vi "main.vi"() -> ()   [LabVIEW 2017]
uses:
  <vilib>/DAQmx/read.llb/DAQmx Read (Counter U32 1Chan 1Samp).vi
  <vilib>/DAQmx/write.llb/DAQmx Write (Digital 1D Bool 1Chan 1Samp).vi
  <vilib>/DAQmx/miscellaneous.llb/DAQmx Fill In Error Info.vi
panel:
  in  "Digital real/sham stim channels":tag="pciDAQ/port0/line1:2"
  in  "Analog pulse channel":tag="pciDAQ/ao0"
  in  "OEP sample clock in":tag="/pciDAQ/PFI0"
  in  "Onboard counter":tag="pciDAQ/ctr0"
  out "Learning rate (for adaptive threshold)":dbl(graph)
  out "Phase threshold":sgl(graph)
  in  "Stim even when\ntarget exceeded":bool=TRUE
  in  "Sham stimulations:":i32=1 min=0
  in  "Real stimulations:":i32=1 min=1
  out "Stim time":i64
  out "Crossing time":i64
  out "Crossing level":sgl
  out "Time on (samp.)":i64
  out "Clock offset":i64
  in  "OEP stim TTL chan":u16=4 caption="probe channel" min=1 max=8
  in  "event channel":u16=1 min=1 max=8
  in  "event port":u16=5557
  out "New event":bool
  in  "Max target":i64 min=0
  in  "Limit target":bool
  in  "Target delay":i64
  in  "Adapt target":bool
  out "Phase offset (deg.)":dbl
  in  "Avg signal freq (Hz)":dbl=6.0
  in  "Sample rate":dbl=30000.0
  in  "Stim enabled":bool
  out "OEP to LV delay":i64(graph)=402
  in  "Stop":bool
  # "*** Start OpenEphys acquisition before the VI. ***"
  # "*** In the audio settings in the OpenEphys GUI, reduce the buffer size to get a 10 ms buffer period.  If ASIO is installed and enabled in\nthe Open Ephys build, use ASIO with sample rate (in audio settings) = 192,000 Hz and buffer size = 192 (1 ms buffer period). ***"
  # "Inputs"
  # "Delay control"
  # "Stim pattern if enabled"
  # "Event info"
  # "Threshold estimation"
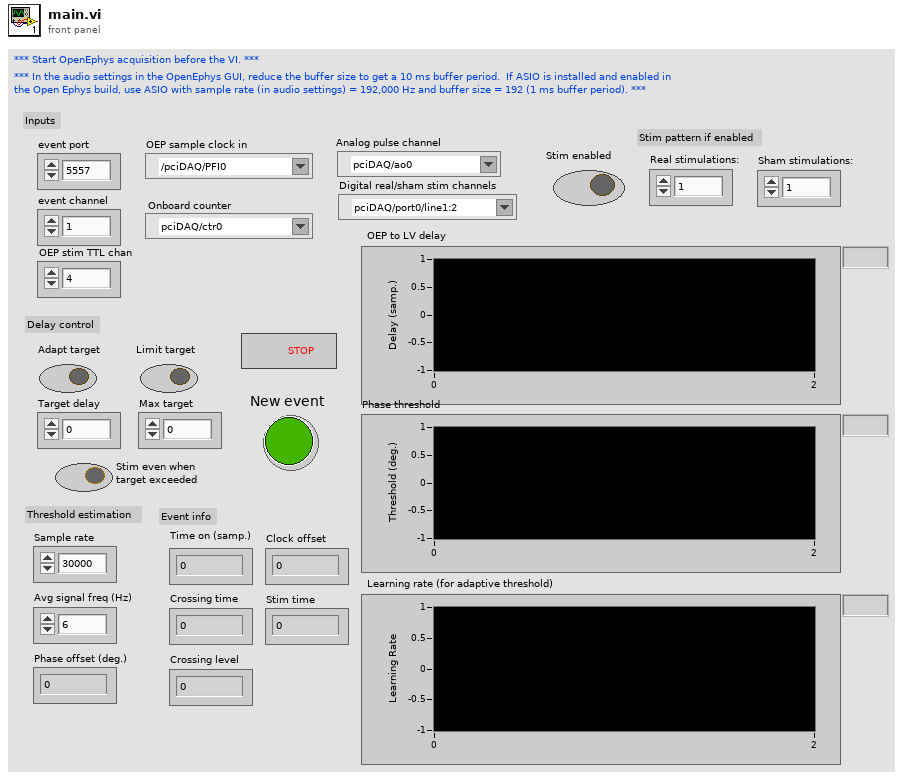
[diagram p1: front panel]
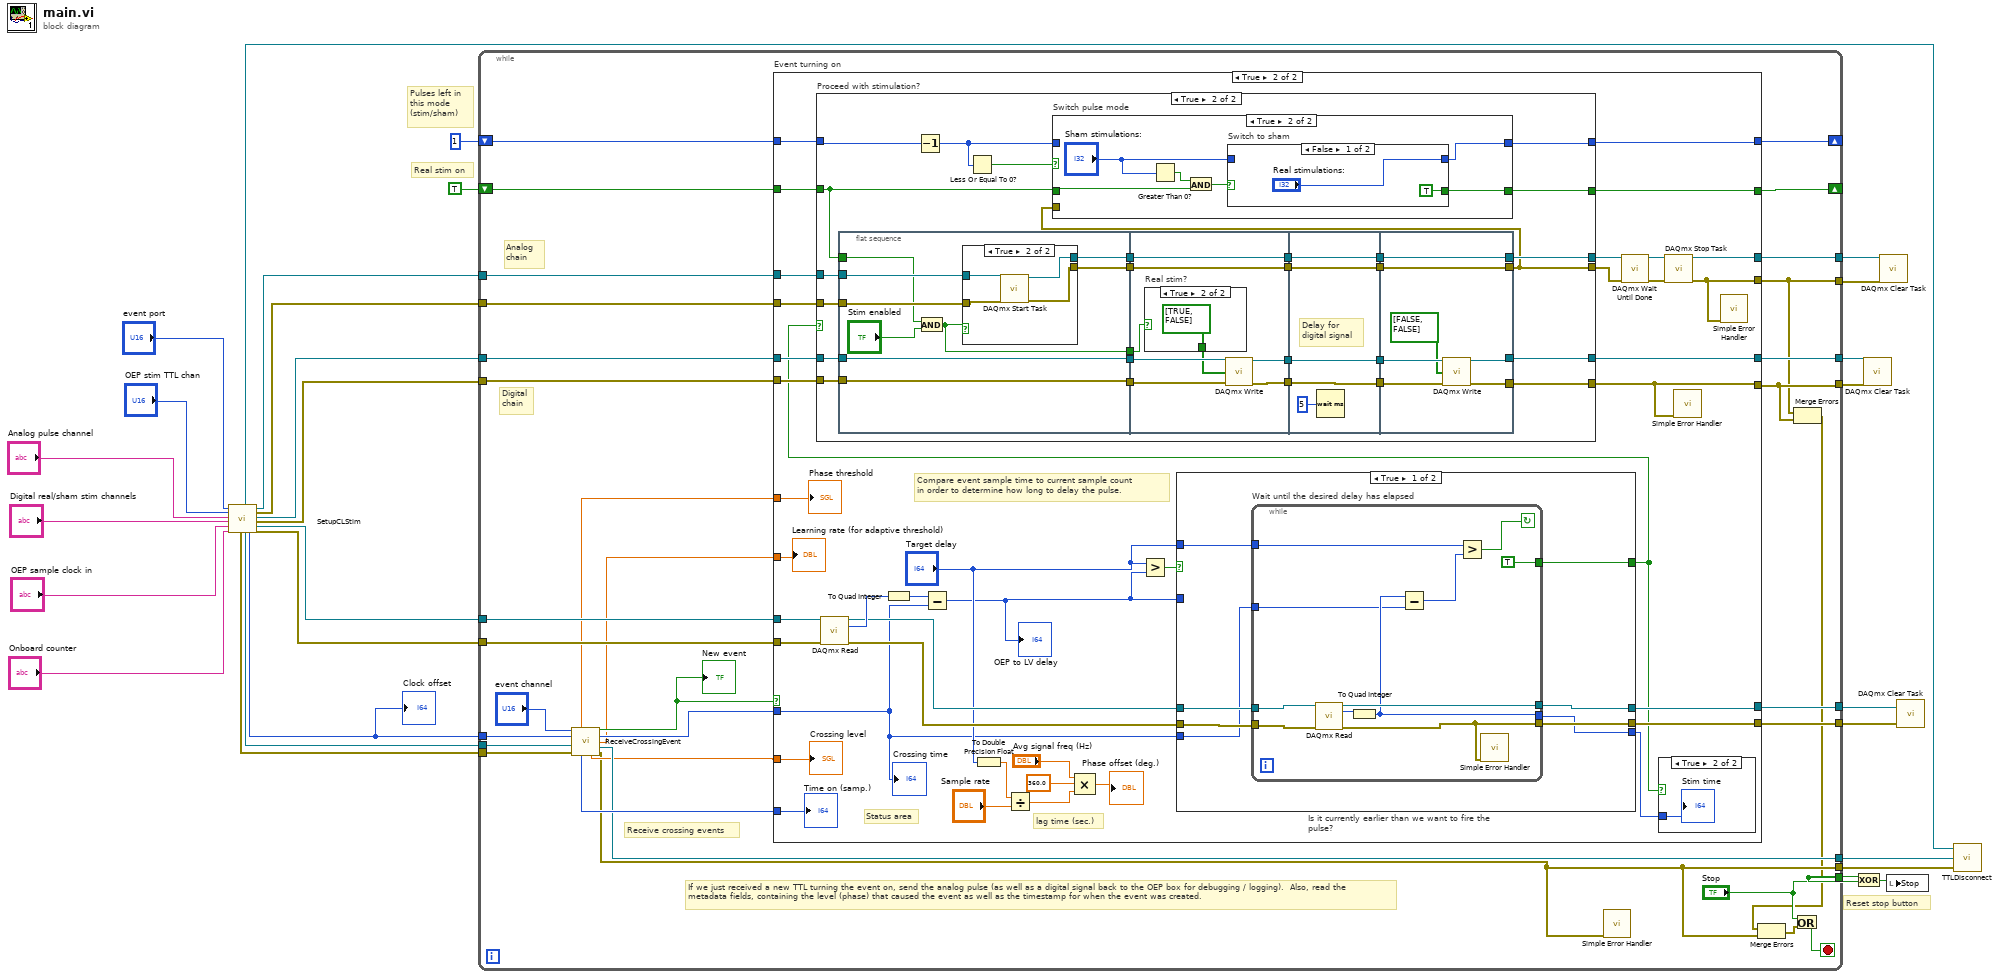
[diagram p0: block diagram]
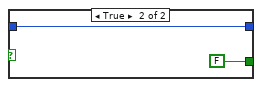
[diagram p6: hidden frame]
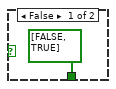
[diagram p8: hidden frame]
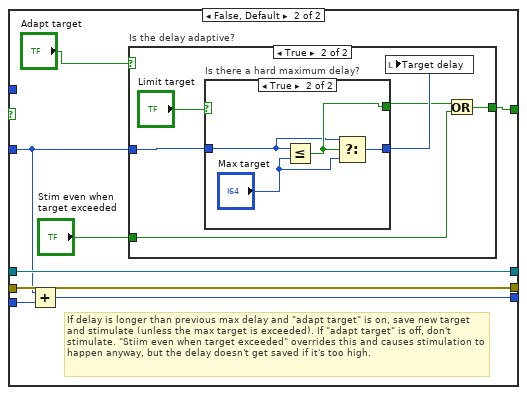
[diagram p9: hidden frame]
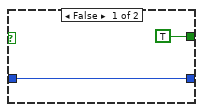
[diagram p11: hidden frame]
diagram:
  # "Pulses left in \nthis mode\n(stim/sham)"
  # "Real stim on"
  # "Reset stop button"
  n1 = call "SetupCLStim.vi"("event port"="event port", "OEP pulse channel"="OEP stim TTL chan", "Analog pulse channel"="Analog pulse channel", "Digital real/sham stim channels"="Digital real/sham stim channels", "OEP sample clock in"="OEP sample clock in", "Onboard counter"="Onboard counter") -> ("zmq error out"=w7:errorcluster, "context out"=w16:refnum<class "zmq_context.lvclass">, "socket out"=w8:refnum<class "zmq_socket.lvclass">, "clock offset"=w9:i64, "AO task out"=w15:refnum<k21>, "AO error out"=w14:errorcluster, "DO task out"=w13:refnum<k21>, "DO error out"=w12:errorcluster, "ctr task out"=w11:refnum<k21>, "ctr error out"=w10:errorcluster)  [unwired: 4 in]
  "Clock offset" <- w9
  n2 = while {
    tunnel: w7 -> [w49]
    tunnel: [w32] -> w24
    tunnel: w8 -> [w50]
    tunnel: w15 -> [w60]
    tunnel: w13 -> [w59]
    tunnel: w12 -> [w58]
    tunnel: w14 -> [w53]
    tunnel: [w51] -> w18
    tunnel: [w31] -> w17
    tunnel: [w57] -> w28
    tunnel: [w33] -> w27
    tunnel: ["Stop"] -> w26
    tunnel: w11 -> [w56]
    tunnel: [w55] -> w23
    tunnel: [w54] -> w22
    tunnel: w10 -> [w52]
    tunnel: [w45] -> w21
    shift-right: [w39] -> _
    shift-left: TRUE -> [w41]
    shift-right: [w40] -> _
    shift-left: 1 -> [w42]
    tunnel: w9 -> [w29]
    stop <- w36 stop-if-true
    # "Analog \nchain"
    # "Digital\nchain"
    # "If we just received a new TTL turning the event on, send the analog pulse (as well as a digital signal back to the OEP box for debugging / logging).  Also, read the metadata fields, containing the level (phase) that caused the event as well as the timestamp for when the event was created."
    # "Receive crossing events"
    n3 = call "ReceiveCrossingEvent.vi"("channel"="event channel", "clock offset"=w29, "socket in"=w50, "error in"=w49) -> ("threshold"=w38:sgl, "new crossing"=w48:bool, "crossing time"=w47:i64, "learning rate"=w37:dbl, "socket out"=w45:refnum<class "zmq_socket.lvclass">, "event time"=w46:i64, "crossing level"=w44:sgl, "error out"=w32:errorcluster)  [unwired: 3 in, 1 out]
    "New event" <- w48
    n4 = case "Event turning on" shown="True" w48 {
      tunnel: w60 -> [w68 w104]
      tunnel: w53 -> [w67 w103]
      tunnel: [w68 w95] -> w51
      tunnel: [w67 w72] -> w31
      tunnel: w59 -> [w66 w107]
      tunnel: w58 -> [w65 w105]
      tunnel: [w66 w108] -> w57
      tunnel: [w65 w71] -> w33
      tunnel: w47 -> [_ w90]
      tunnel: w56 -> [w64 w102]
      tunnel: w52 -> [w63 w99]
      tunnel: [w64 w97] -> w55
      tunnel: [w63 w96] -> w54
      tunnel: w46 -> [_ w91]
      tunnel: w44 -> [_ w85]
      tunnel: w42 -> [w62 w78]
      tunnel: w41 -> [w61 w77]
      tunnel: [w62 w76] -> w40
      tunnel: [w61 w75] -> w39
      tunnel: w38 -> [_ w74]
      tunnel: w37 -> [_ w73]
      frame False {
      }
      frame True {
        # "Status area"
        # "lag time (sec.)"
        # "Compare event sample time to current sample count\nin order to determine how long to delay the pulse."
        n5 = call-poly <vilib>:"DAQmx Read.vi"("task/channels in"=w102, "error in"=w99) -> ("task out"=w98:refnum<k21>, "data"=w101:u32, "error out"=w100:errorcluster)  [unwired: 11 in]
        n6 = To Quad Integer(1:w101) -> (0:w81:i64)
        n7 = Subtract(x=w81, y=w90) -> (x-y=w92:i64)
        "OEP to LV delay" <- w92
        n8 = To Double Precision Float(number="Target delay") -> (double precision float=w89:dbl)
        n9 = Divide(x=w89, y="Sample rate") -> (x/y=w88:dbl)
        n10 = Compound Arithmetic op=MULTIPLY("Avg signal freq (Hz)", 360.0 ("y"), w88) -> (→"Phase offset (deg.)":dbl)
        n11 = Greater?(x="Target delay", y=w92) -> (0:w106:bool)
        n12 = case "Is it currently earlier than we want to fire the pulse?" shown="True" w106 {
          tunnel: w92 -> [_ w213]
          tunnel: "Target delay" -> [w193 _]
          tunnel: w100 -> [w198 w218]
          tunnel: [w197 w218] -> w96
          tunnel: w90 -> [w192 w216]
          tunnel: w98 -> [w199 w217]
          tunnel: [w196 w217] -> w97
          tunnel: [w195 w212] -> w80
          tunnel: [w194 w215] -> w79
          frame True {
            n13 = while "Wait until the desired delay has elapsed" {
              tunnel: w199 -> [w209]
              tunnel: w198 -> [w210]
              tunnel: [w200] -> w197
              tunnel: [w208] -> w196
              tunnel: [TRUE] -> w195
              tunnel: [w203] -> w194
              tunnel: w193 -> [w204]
              tunnel: w192 -> [w202]
              stop <- w206 continue-if-true
              n14 = call-poly <vilib>:"DAQmx Read.vi"("task/channels in"=w209, "error in"=w210) -> ("task out"=w208:refnum<k21>, "data"=w205:u32, "error out"=w200:errorcluster)  [unwired: 11 in]
              n15 = To Quad Integer(1:w205) -> (0:w203:i64)
              n16 = Subtract(x=w203, y=w202) -> (x-y=w201:i64)
              n17 = Greater?(x=w204, y=w201) -> (0:w206:bool)
              n18 = call <vilib>:"Simple Error Handler.vi"("error in (no error)"=w200) -> ()  [unwired: 4 in, 5 out]
            }
          }
          frame False, Default {
            # "If delay is longer than previous max delay and \"adapt target\" is on, save new target and stimulate (unless the max target is exceeded). If \"adapt target\" is off, don't stimulate. \"Stiim even when target exceeded\" overrides this and causes stimulation to happen anyway, but the delay doesn't get saved if it's too high."
            n19 = Add(x=w213, y=w216) -> (x+y=w215:i64)
            n20 = case "Is the delay adaptive?" shown="True" "Adapt target" {
              tunnel: w213 -> [_ w224]
              tunnel: [w219 w222] -> w212
              tunnel: "Stim even when\ntarget exceeded" -> [w219 w220]
              frame False {
              }
              frame True {
                n21 = case "Is there a hard maximum delay?" shown="True" "Limit target" {
                  tunnel: [w227 w231] -> w223
                  tunnel: w224 -> [w227 w229]
                  tunnel: [TRUE w230] -> w221
                  frame False {
                  }
                  frame True {
                    n22 = Less Or Equal?(x=w229, y="Max target") -> (x <= y?=w230:bool)
                    n23 = Select(t=w229, s=w230, f="Max target") -> (s? t:f=w231:i64)
                  }
                }
                n24 = local write "Target delay"(w223) -> ()
                n25 = Or(x=w221, y=w220) -> (x .or. y?=w222:bool)
              }
            }
          }
        }
        n26 = case "Proceed with stimulation?" shown="True" w80 {
          tunnel: [w113 w130] -> w108
          tunnel: w107 -> [w113 w129]
          tunnel: w105 -> [w112 w128]
          tunnel: w104 -> [w115 w127]
          tunnel: w103 -> [w114 w126]
          tunnel: [w112 w125] -> w71
          tunnel: [w114 w122] -> w82
          tunnel: [w115 w124] -> w94
          tunnel: w78 -> [w111 w121]
          tunnel: w77 -> [w110 w118]
          tunnel: [w111 w117] -> w76
          tunnel: [w110 w116] -> w75
          frame False {
          }
          frame True {
            n27 = flat-sequence {
              tunnel: [w163] -> w142
              tunnel: [w160] -> w141
              tunnel: [w159] -> w140
              tunnel: w128 -> [w159]
              tunnel: w129 -> [w160]
              tunnel: w126 -> [w162]
              tunnel: w127 -> [w161]
              tunnel: [w158] -> w139
              tunnel: w118 -> [w156]
              tunnel: [w155] -> w123
              tunnel: [w175] -> w138
              tunnel: [w173] -> w137
              tunnel: w142 -> [w177]
              tunnel: [w177] -> w136
              tunnel: w141 -> [w176]
              tunnel: w140 -> [w174]
              tunnel: w139 -> [w172]
              tunnel: [w172] -> w135
              tunnel: w123 -> [w171]
              tunnel: [w184] -> w134
              tunnel: w138 -> [w184]
              tunnel: [w183] -> w133
              tunnel: w137 -> [w183]
              tunnel: w136 -> [w181]
              tunnel: [w181] -> w132
              tunnel: w135 -> [w180]
              tunnel: [w180] -> w131
              tunnel: [w190] -> w130
              tunnel: w134 -> [w191]
              tunnel: w133 -> [w189]
              tunnel: [w188] -> w125
              tunnel: w132 -> [w187]
              tunnel: [w187] -> w124
              tunnel: [w186] -> w122
              tunnel: w131 -> [w186]
              frame #0 {
                n28 = And(x=w156, y="Stim enabled") -> (x .and. y?=w155:bool)
                n29 = case shown="True" w155 {
                  tunnel: [w165 w169] -> w163
                  tunnel: w162 -> [w164 w168]
                  tunnel: w161 -> [w165 w167]
                  tunnel: [w164 w166] -> w158
                  frame False {
                  }
                  frame True {
                    n30 = call <vilib>:"DAQmx Start Task.vi"("task/channels in"=w167, "error in"=w168) -> ("task out"=w169:refnum<k21>, "error out"=w166:errorcluster)  [unwired: 12 in]
                  }
                }
              }
              frame #1 {
                n31 = case "Real stim?" shown="True" w171 {
                  tunnel: [bool[] [FALSE, TRUE] ("data") bool[] [TRUE, FALSE] ("data")] -> w170
                  frame False {
                  }
                  frame True {
                  }
                }
                n32 = call-poly <vilib>:"DAQmx Write.vi"("task/channels in"=w176, "data"=w170, "error in"=w174) -> ("task out"=w175:refnum<k21>, "error out"=w173:errorcluster)  [unwired: 10 in, 1 out]
              }
              frame #2 {
                # "Delay for \ndigital signal"
                n33 = Wait (ms)(milliseconds to wait=u32 5) -> ()  [unwired: 1 out]
              }
              frame #3 {
                n34 = call-poly <vilib>:"DAQmx Write.vi"("task/channels in"=w191, "data"=bool[] [FALSE, FALSE], "error in"=w189) -> ("task out"=w190:refnum<k21>, "error out"=w188:errorcluster)  [unwired: 10 in, 1 out]
              }
            }
            n35 = Decrement(x=w121) -> (x-1=w119:i32)
            n36 = Less Or Equal To 0?(x=w119) -> (x <= 0?=w120:bool)
            n37 = case "Switch pulse mode" shown="True" w120 {
              tunnel: w122 -> [_ _]
              tunnel: w119 -> [w144 _]
              tunnel: w118 -> [w143 w149]
              tunnel: [w144 w146] -> w117
              tunnel: [w143 w145] -> w116
              frame False {
              }
              frame True {
                n38 = Greater Than 0?(x="Sham stimulations:") -> (x > 0?=w150:bool)
                n39 = And(x=w150, y=w149) -> (x .and. y?=w148:bool)
                n40 = case "Switch to sham" shown="False" w148 {
                  tunnel: "Sham stimulations:" -> [_ w154]
                  tunnel: ["Real stimulations:" w154] -> w146
                  tunnel: [TRUE FALSE] -> w145
                  frame False {
                  }
                  frame True {
                  }
                }
              }
            }
          }
        }
        n41 = call <vilib>:"DAQmx Wait Until Done.vi"("task/channels in"=w94, "error in"=w82) -> ("task out"=w69:refnum<k21>, "error out"=w70:errorcluster)  [unwired: 12 in]
        n42 = case shown="True" w80 {
          tunnel: w79 -> [_ w109]
          frame False {
          }
          frame True {
            "Stim time" <- w109
          }
        }
        n43 = call <vilib>:"DAQmx Stop Task.vi"("task/channels in"=w69, "error in"=w70) -> ("task out"=w95:refnum<k21>, "error out"=w72:errorcluster)  [unwired: 12 in]
        n44 = call <vilib>:"Simple Error Handler.vi"("error in (no error)"=w71) -> ()  [unwired: 4 in, 5 out]
        n45 = call <vilib>:"Simple Error Handler.vi"("error in (no error)"=w72) -> ()  [unwired: 4 in, 5 out]
        "Time on (samp.)" <- w91
        "Crossing time" <- w90
        "Crossing level" <- w85
        "Phase threshold" <- w74
        "Learning rate (for adaptive threshold)" <- w73
      }
    }
    n46 = call <vilib>:"Simple Error Handler.vi"("error in (no error)"=w32) -> ()  [unwired: 4 in, 5 out]
    n47 = Merge Errors(w31, w33) -> (w30:errorcluster)
    n48 = Merge Errors(w30, w32) -> (w34:errorcluster)
    n49 = Or(x="Stop", y=w34) -> (x .or. y?=w36:bool)
  }
  n50 = Exclusive Or(1:w26, 2:w26) -> (0:w25:bool)
  n51 = call <vilib>:"DAQmx Clear Task.vi"("task in"=w28, "error in"=w27) -> ()  [unwired: 13 in, 1 out]
  n52 = call <vilib>:"DAQmx Clear Task.vi"("task in"=w18, "error in"=w17) -> ()  [unwired: 13 in, 1 out]
  n53 = local write "Stop"(w25) -> ()
  n54 = call <vilib>:"DAQmx Clear Task.vi"("task in"=w23, "error in"=w22) -> ()  [unwired: 13 in, 1 out]
  n55 = call "TTLDisconnect.vi"("error in"=w24, "socket in"=w21, "context in"=w16) -> ()  [unwired: 1 in, 1 out]
